vi "Generate tmp points.vi"(8 "Type":enum16{"Log", "Quadratic", "Cubic", "Linear"}(ring), 9 "Number of points":i32=100, 10 "End point":dbl=280.0, 11 "Start point":dbl=302.0) -> (3 "Array":dbl[](array[numeric]))   [LabVIEW 2021]
uses:
  <vilib>/Analysis/1siggen.llb/Ramp Pattern by Samples.vi
  <vilib>/Analysis/NI_AALBase.lvlib
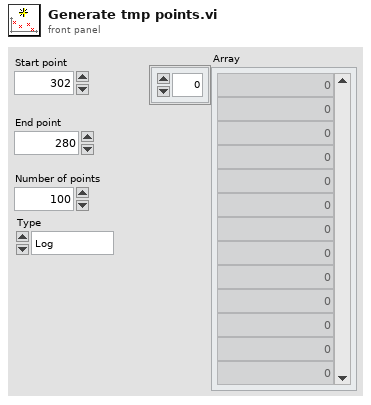
[diagram p1: front panel]
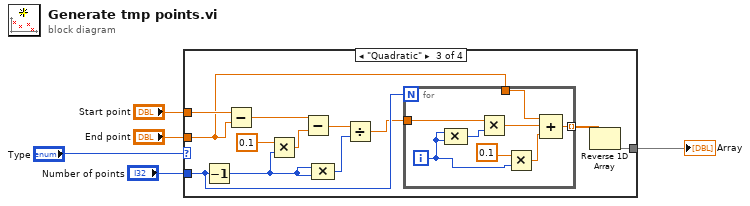
[diagram p0: block diagram]
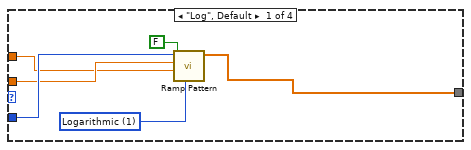
[diagram p2: hidden frame]
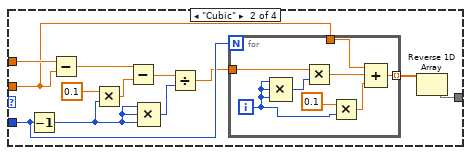
[diagram p3: hidden frame]
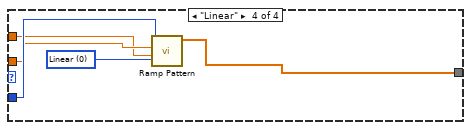
[diagram p4: hidden frame]
diagram:
  n1 = case shown="\"Quadratic\"" "Type" {
    tunnel: [w6 w12 w32 w55] -> w5
    tunnel: "Number of points" -> [w10 w20 w40 w54]
    tunnel: "End point" -> [w9 w19 w39 w53]
    tunnel: "Start point" -> [w8 w23 w43 w52]
    frame "Log", Default {
      w11 = u16 1 items=["Linear", "Logarithmic"] ("type")
      n2 = call-poly <vilib>:"Ramp Pattern.vi"("type"=w11, "exclude end?"=FALSE, "start"=w8, "end"=w9, "samples"=w10) -> ("Ramp Pattern"=w6:dbl[])  [unwired: 5 in, 1 out]
    }
    frame "Cubic" {
      n3 = Decrement(x=w20) -> (x-1=w15:i32)
      n4 = Subtract(x=w23, y=w19) -> (x-y=w22:dbl)
      n5 = Multiply(x=0.1, y=w15) -> (x*y=w16:dbl)
      n6 = Subtract(x=w22, y=w16) -> (x-y=w17:dbl)
      n7 = Compound Arithmetic op=MULTIPLY(w15, w15, w15) -> (w21:i32)
      n8 = Divide(x=w17, y=w21) -> (x/y=w18:dbl)
      n9 = for {
        N: w20 -> [_]
        tunnel: w19 -> [w30]
        tunnel: [w31] -> w13 mode=indexing
        tunnel: w18 -> [w27]
        i -> [w24]
        n10 = Compound Arithmetic op=MULTIPLY(w24, w24, w24) -> (w28:i32)
        n11 = Multiply(x=w27, y=w28) -> (x*y=w29:dbl)
        n12 = Multiply(x=0.1, y=w24) -> (x*y=w26:dbl)
        n13 = Compound Arithmetic op=ADD(w30, w29, w26) -> (w31:dbl)
      }
      n14 = Reverse 1D Array(array=w13) -> (reversed array=w12:dbl[])
    }
    frame "Quadratic" {
      n15 = Decrement(x=w40) -> (x-1=w35:i32)
      n16 = Subtract(x=w43, y=w39) -> (x-y=w42:dbl)
      n17 = Multiply(x=0.1, y=w35) -> (x*y=w36:dbl)
      n18 = Subtract(x=w42, y=w36) -> (x-y=w37:dbl)
      n19 = Compound Arithmetic op=MULTIPLY(w35, w35) -> (w41:i32)
      n20 = Divide(x=w37, y=w41) -> (x/y=w38:dbl)
      n21 = for {
        N: w40 -> [_]
        tunnel: w39 -> [w50]
        tunnel: [w51] -> w33 mode=indexing
        tunnel: w38 -> [w47]
        i -> [w44]
        n22 = Compound Arithmetic op=MULTIPLY(w44, w44) -> (w48:i32)
        n23 = Multiply(x=w47, y=w48) -> (x*y=w49:dbl)
        n24 = Multiply(x=0.1, y=w44) -> (x*y=w46:dbl)
        n25 = Compound Arithmetic op=ADD(w50, w49, w46) -> (w51:dbl)
      }
      n26 = Reverse 1D Array(array=w33) -> (reversed array=w32:dbl[])
    }
    frame "Linear" {
      w56 = u16 0 items=["Linear", "Logarithmic"] ("type")
      n27 = call-poly <vilib>:"Ramp Pattern.vi"("type"=w56, "start"=w52, "end"=w53, "samples"=w54) -> ("Ramp Pattern"=w55:dbl[])  [unwired: 6 in, 1 out]
    }
  }
  "Array" <- w5
